vi "Larger window user menu handler.vi"(9 "Image":T1, 10 "ItemTag":string, 11 "Window VI's Ref":refnum<vi>) -> ()   [LabVIEW 2013]
uses:
  <vilib>/vision/Image Controls.llb/IMAQ Image.ctl
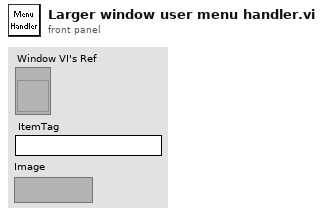
[diagram p1: front panel]
types:
  T1 = typedef "IMAQ Image.ctl" = refnum<image>
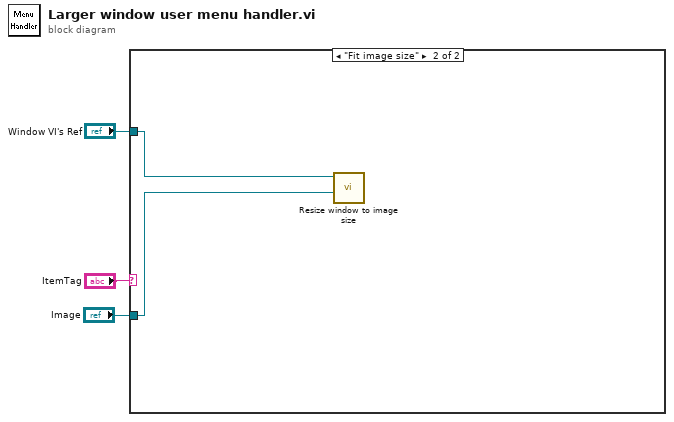
[diagram p0: block diagram]
diagram:
  n1 = case shown="\"Fit image size\"" "ItemTag" {
    tunnel: "Image" -> [_ w5]
    tunnel: "Window VI's Ref" -> [_ w4]
    frame Default {
    }
    frame "Fit image size" {
      n2 = call "Resize window to image size.vi"("Image"=w5, "Window VI's Ref"=w4) -> ()  [unwired: 10 in]
    }
  }
